vi "example_01_wait.vi"() -> ()   [LabVIEW 2015, in "lv-waitgroup.lvlib"]
uses:
  lv-waitgroup.lvlib
panel:
  in  "timeout_ms":i32
  out "error out":errorcluster
  in  "skip_done":bool
  in  "queue_size":i32=5
  out "processes_remaining []":i32[](array[numeric])
  out "active":i32
  in  "wait_time_ms":u32=5000
  in  "stop":bool
  in  "do_it_button":bool
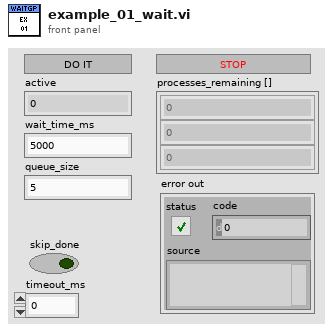
[diagram p1: front panel]
types:
  T1 = typedef "lv-waitgroup.lvlib/api_waitgroup.ctl" = string
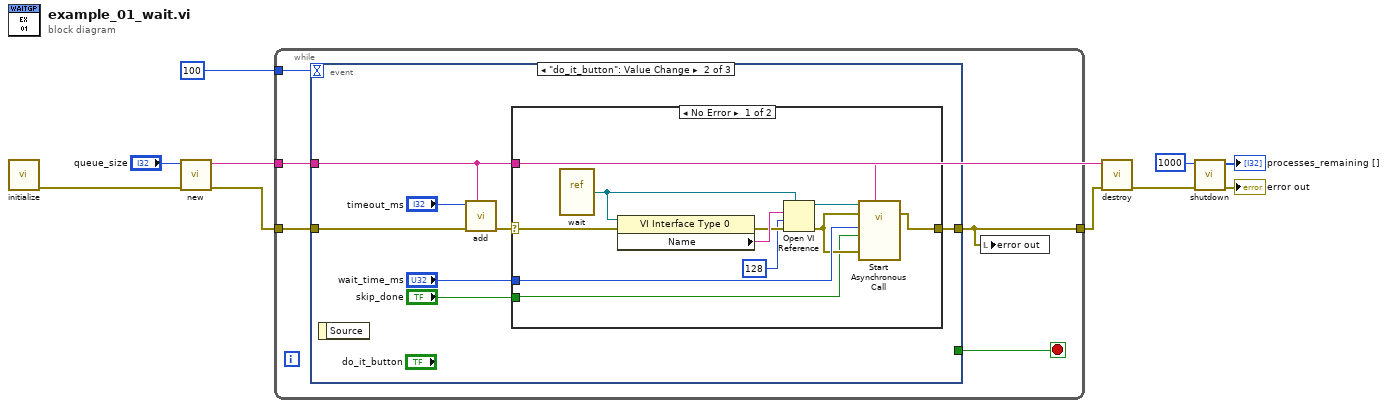
[diagram p0: block diagram]
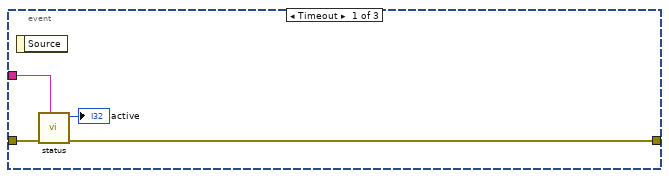
[diagram p2: hidden frame]
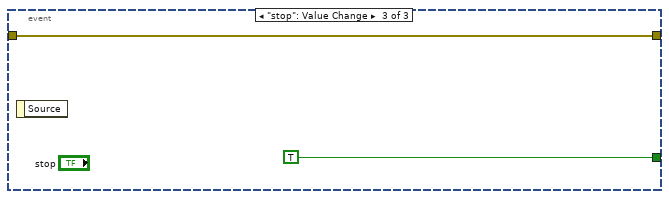
[diagram p4: hidden frame]
diagram:
  n1 = call "initialize.vi"() -> ("error out"=w9:errorcluster)  [unwired: 11 in]
  n2 = call "new.vi"("error in (no error)"=w9, "queue_size"="queue_size") -> ("error out"=w8:errorcluster, "waitgroup"=w5:T1)  [unwired: 8 in]
  n3 = while {
    tunnel: 100 -> [w14]
    tunnel: w8 -> [w13]
    tunnel: [w11] -> w7
    tunnel: w5 -> [w12]
    stop <- w15 stop-if-true
    n4 = event shown="[1] \"do_it_button\": Value Change" {
      selector: _ -> [_ _ _]
      dyn-events: _ -> [_ _ _]
      timeout: w14 -> [_ _ _]
      tunnel: [_ _ TRUE] -> w15
      tunnel: w13 -> [w18 w24 w39]
      tunnel: [w17 w25 w39] -> w11
      tunnel: w12 -> [w16 w22 _]
      event Timeout {
        n5 = event-data() -> ()  [unwired: 1 in, 1 out]
        n6 = call "status.vi"("waitgroup"=w16, "error in (no error)"=w18) -> ("error out"=w17:errorcluster, "active"=→"active":i32)  [unwired: 8 in]
      }
      event "do_it_button": Value Change {
        n7 = event-data() -> ()  [unwired: 1 in, 1 out]
        n8 = call "add.vi"("waitgroup"=w22, "error in (no error)"=w24, "timeout_ms"="timeout_ms") -> ("error out"=w23:errorcluster)  [unwired: 8 in]
        n9 = case shown="No Error" w23 {
          selector: w23 -> [w30 w38]
          tunnel: "wait_time_ms" -> [w32 _]
          tunnel: [w31 w38] -> w25
          tunnel: w22 -> [w29 _]
          tunnel: "skip_done" -> [w27 _]
          frame No Error {
            n10 = vi-ref "wait.vi"() -> (w36:refnum<vi>)
            n11 = property class="VI Interface Type 0"(reference=w36, error in=w30) -> (error out=w35:errorcluster, "Name"=w37:string)  [unwired: 1 out]
            n12 = Open VI Reference(type specifier VI Refnum (for type only)=w36, vi path=w37, options=128, error in (no error)=w35) -> (vi reference=w34:refnum<vi>, error out=w28:errorcluster)  [unwired: 2 in]
            n13 = call-by-ref "Start Asynchronous Call"(reference=w34, error in=w28, "waitgroup"=w29, 8:"error in (no error)"=w28, "skip_done"=w27, "wait_ms"=w32) -> (error out=w31:errorcluster)  [unwired: 7 in, 2 out]
          }
          frame Error {
          }
        }
      }
      event "stop": Value Change {
        n14 = event-data() -> ()  [unwired: 1 in, 1 out]
      }
    }
    n15 = local write "error out"(w11) -> ()
  }
  n16 = call "destroy.vi"("error in (no error)"=w7, "waitgroup"=w5) -> ("error out"=w6:errorcluster)  [unwired: 8 in, 1 out]
  n17 = call "shutdown.vi"("error in (no error)"=w6, "wait_ms"=1000) -> ("error out"=→"error out":errorcluster, "processes_remaining []"=→"processes_remaining []":i32[])  [unwired: 8 in]
